vi "VerifOnePos.vi"() -> ()   [LabVIEW 2018]
panel:
  out "One position":bool
  in  "sequencias":u16
  out "log2(x)":dbl
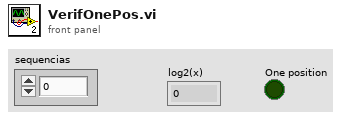
[diagram p1: front panel]
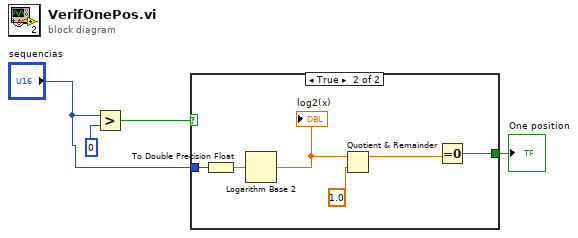
[diagram p0: block diagram]
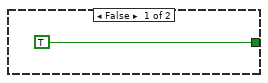
[diagram p2: hidden frame]
diagram:
  n1 = Greater?(x="sequencias", y=u16 0) -> (0:w1:bool)
  n2 = case shown="True" w1 {
    tunnel: [TRUE w8] -> w4
    tunnel: "sequencias" -> [_ w11]
    frame False {
    }
    frame True {
      n3 = To Double Precision Float(number=w11) -> (double precision float=w10:dbl)
      n4 = Logarithm Base 2(1:w10) -> (0:w6:dbl)
      "log2(x)" <- w6
      n5 = Quotient & Remainder(x=w6, y=1.0) -> (x-y*floor(x/y)=w9:dbl)  [unwired: 1 out]
      n6 = Equal To 0?(x=w9) -> (x = 0?=w8:bool)
    }
  }
  "One position" <- w4
